vi "ReadCmdIn.vi"(0 "Connections":T1(array[cluster]), 2 "Log in":T2[](array[typedef]), 3 "Err in":string) -> (4 "data":string, 5 "Connections out":T1(array[cluster]), 6 "Log out":T2[](array[typedef]), 7 "Err out":string)   [LabVIEW 2012]
uses:
  ROSLog.ctl
  _ROSDefinition.vi
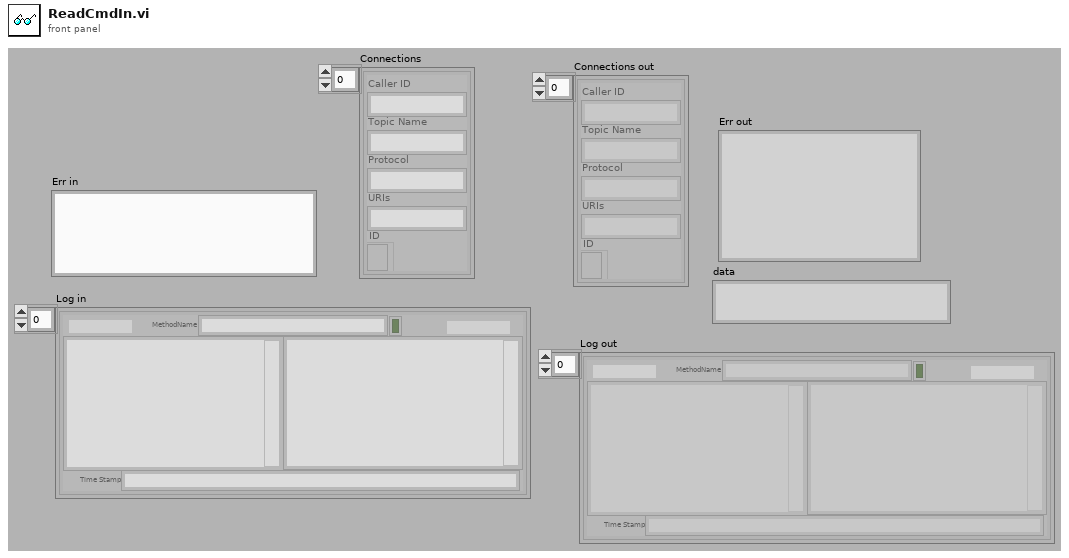
[diagram p1: front panel]
types:
  T1 = cluster{"Caller ID":string, "Topic Name":string, "Protocol":string, "URIs":string, "ID":refnum<k5>}[]
  T2 = typedef "ROSLog.ctl" = cluster{"Sent":string, "Reply":string, "MethodName":string, "success":bool, "Dir1":string, "Dir2":string, "Time Stamp":string}
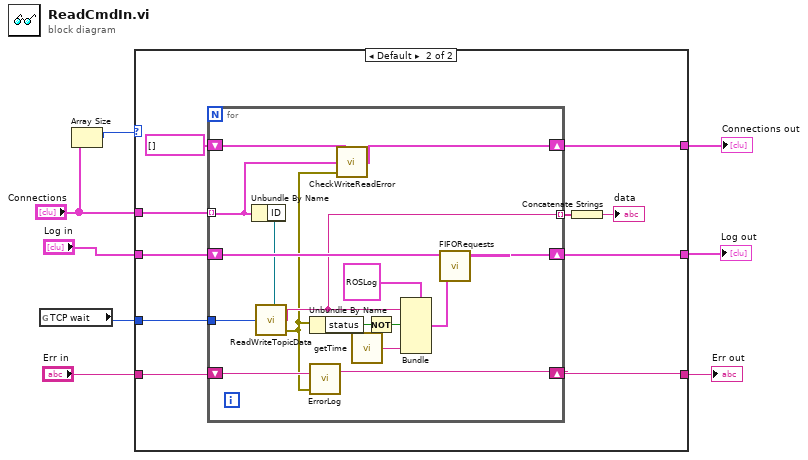
[diagram p0: block diagram]
diagram:
  n1 = global read "_ROSDefinition.vi" "TCP wait"() -> (w1:i32)
  n2 = Array Size(array="Connections") -> (size(s)=w3:i32)
  n3 = case shown="Default" w3 {
    tunnel: [w11 w21] -> w8
    tunnel: "Log in" -> [w11 w20]
    tunnel: "Err in" -> [w10 w19]
    tunnel: [w10 w18] -> w5
    tunnel: "Connections" -> [w9 w17]
    tunnel: [w9 w14] -> w2
    tunnel: w1 -> [_ w12]
    frame 0 {
    }
    frame Default {
      n4 = for {
        shift-right: [w37] -> w18
        shift-left: w19 -> [w36]
        shift-right: [w30] -> w21
        shift-left: w20 -> [w31]
        tunnel: w17 -> [w26] mode=indexing
        tunnel: [w28] -> w16 mode=indexing
        shift-right: [w24] -> w14
        shift-left: T1 [] ("Connections out") -> [w23]
        tunnel: w12 -> [w22]
        n5 = Unbundle By Name(w26) -> ("ID"=w29:refnum<k5>)
        n6 = call "ReadWriteTopicData.vi"("timeout ms (1000)"=w22, "connection ID in"=w29) -> ("error out"=w25:errorcluster, "data out"=w28:string)  [unwired: 1 in, 1 out]
        n7 = Unbundle By Name(w25) -> ("status"=w33:bool)
        n8 = call "ErrorLog.vi"("error in"=w25, "String in"=w36) -> ("String out"=w37:string)  [unwired: 1 in, 1 out]
        n9 = call "CheckWriteReadError.vi"("error"=w25, "Subscriber in"=w26, "Connections in"=w23) -> ("Connections out"=w24:T1)
        n10 = call "getTime.vi"() -> ("Current Time"=w35:string)  [unwired: 1 in]
        n11 = Not(x=w33) -> (.not. x?=w32:bool)
        n12 = Bundle(cluster=T2 {"Sent"="", "Reply"="", "MethodName"="read", "success"=FALSE, "Dir1"="To ROS", "Dir2"="From ROS", "Time Stamp"=""} ("Log"), "Reply"=w28, "success"=w32, "Time Stamp"=w35) -> (w34:T2)  [unwired: 4 in]
        n13 = call "FIFORequests.vi"("Log"=w34, "Requests in"=w31) -> ("Requests out"=w30:T2[])  [unwired: 1 in]
      }
      n14 = Concatenate Strings(w16) -> (→"data":string)
    }
  }
  "Log out" <- w8
  "Err out" <- w5
  "Connections out" <- w2
